vi "UHR-Fleezers Control (host) - 16.2.2v2.vi"() -> ()   [LabVIEW 2014] (continued)
                n1050 = Add(x=w1636, y=w1632) -> (x+y=w1628:dbl)
                n1051 = Greater Or Equal?(x=w1628, y=w1629) -> (x >= y?=w1630:bool)
                n1052 = Select(t=w1629, s=w1630, f=w1628) -> (s? t:f=w1624:dbl)
                n1053 = Index Array(array=w1627, index=1) -> (element=w1625:dbl)
                n1054 = Greater?(x=w1623, y=0) -> (0:w1618:bool)
                n1055 = Greater Or Equal?(x=w1628, y=w1625) -> (x >= y?=w1643:bool)
                n1056 = Select(t=w1618, s="No pause on first pull", f=TRUE ("Scanning (slow scan)")) -> (s? t:f=w1620:bool)
                n1057 = Compound Arithmetic op=AND(w1643, "Stop at pause on pull", w1639, w1620) -> (w1642:bool)
                n1058 = Compound Arithmetic op=OR(w1630, "Immediately quit scan", "Stop pulling and reverse") -> (w1645:bool)
                n1059 = case shown="True" w1642 {
                  tunnel: [w1649 w1651] -> w1640
                  tunnel: w1639 -> [w1649 _]
                  tunnel: w1625 -> [_ w1650]
                  tunnel: w1624 -> [w1648 _]
                  frame False {
                    # "use the current position or the exact position for the final location"
                    n1060 = property on="Trap Delta (MHz)" class="DigNum (strict)"("Val(Sgnl)"=w1648) -> ()  [unwired: 2 in, 2 out]
                  }
                  frame True {
                    # "use the exact postion for the pause"
                    n1061 = while {
                      tunnel: [FALSE] -> w1651
                      i -> [w1662]
                      stop <- w1659 stop-if-true
                      w1663 = u32 100 ("milliseconds to wait")
                      n1062 = local read "Trap pause durations (s)"() -> (w1653:dbl[])
                      n1063 = local read "Immediately quit scan"() -> (w1655:bool)
                      n1064 = Multiply(x="Duration 2 (s)", y=1000.0) -> (x*y=w1664:dbl)
                      n1065 = Divide(x=w1664, y=w1663) -> (x/y=w1661:dbl)
                      n1066 = Wait (ms)(milliseconds to wait=w1663) -> ()  [unwired: 1 out]
                      n1067 = Greater Or Equal?(x=w1662, y=w1661) -> (x >= y?=w1660:bool)
                      n1068 = Or(x="Cancel pause", y=w1655) -> (x .or. y?=w1656:bool)
                      n1069 = Index Array(array=w1653, index=1) -> ()  [unwired: 1 out]
                      n1070 = Or(x=w1660, y=w1656) -> (x .or. y?=w1659:bool)
                    }
                    n1071 = property on="Trap Delta (MHz)" class="DigNum (strict)"("Val(Sgnl)"=w1650) -> ()  [unwired: 2 in, 2 out]
                  }
                }
                "Scanning (slow scan) 2" <- TRUE ("Scanning (slow scan)")
              }
            }
            frame #1 {
              # "Pause between pull/relax"
              # "If you reverse, skip this pause"
              n1072 = Not(x=w1666) -> (.not. x?=w1667:bool)
              n1073 = And(x="Pause after pull, before next relax", y=w1667) -> (x .and. y?=w1668:bool)
              n1074 = case shown="True" w1668 {
                frame False {
                }
                frame True {
                  n1075 = while {
                    i -> [w1679]
                    stop <- w1676 stop-if-true
                    w1680 = u32 100 ("milliseconds to wait")
                    n1076 = local read "Immediately quit scan"() -> (w1673:bool)
                    n1077 = local read "Duration 2 (s)"() -> (w1670:dbl)
                    n1078 = local read "Trap pause durations (s)"() -> (w1671:dbl[])
                    n1079 = local read "Cancel pause"() -> (w1675:bool)
                    n1080 = Multiply(x=w1670, y=1000.0) -> (x*y=w1681:dbl)
                    n1081 = Divide(x=w1681, y=w1680) -> (x/y=w1678:dbl)
                    n1082 = Wait (ms)(milliseconds to wait=w1680) -> ()  [unwired: 1 out]
                    n1083 = Greater Or Equal?(x=w1679, y=w1678) -> (x >= y?=w1677:bool)
                    n1084 = Or(x=w1675, y=w1673) -> (x .or. y?=w1674:bool)
                    n1085 = Index Array(array=w1671, index=2) -> ()  [unwired: 1 out]
                    n1086 = Or(x=w1677, y=w1674) -> (x .or. y?=w1676:bool)
                  }
                }
              }
            }
            frame #2 {
              # "Relax"
              n1087 = while {
                shift-right: [w1702] -> _
                shift-left: TRUE -> [w1701]
                stop <- w1705 stop-if-true
                n1088 = local read "Trap step increment (MHz) (slow scan) 2"() -> (w1696:dbl)
                n1089 = local read "Trap pause positions (MHz)"() -> (w1685:dbl[])
                n1090 = local read "Trap step dwell (ms) (slow scan) 2"() -> (w1692:dbl)
                n1091 = local write "Cancel pause"(FALSE ("Cancel pause")) -> ()
                n1092 = local read "Pause scan"() -> (w1693:bool)
                n1093 = local read "Trap Delta (MHz)"() -> (w1700:dbl)
                n1094 = Index Array(array=w1685, index=0) -> (element=w1689:dbl)
                n1095 = Select(t=0.0, s=w1693, f=w1696) -> (s? t:f=w1695:dbl)
                n1096 = Wait (ms)(milliseconds to wait=w1692) -> ()  [unwired: 1 out]
                n1097 = Subtract(x=w1700, y=w1695) -> (x-y=w1688:dbl)
                n1098 = Less Or Equal?(x=w1688, y=w1689) -> (x <= y?=w1690:bool)
                n1099 = Index Array(array=w1685, index=1) -> (element=w1684:dbl)
                n1100 = local read "Immediately quit scan"() -> (w1699:bool)
                n1101 = Select(t=w1689, s=w1690, f=w1688) -> (s? t:f=w1687:dbl)
                n1102 = Less Or Equal?(x=w1688, y=w1684) -> (x <= y?=w1704:bool)
                n1103 = Compound Arithmetic op=AND(w1704, "Stop at pause on relax", w1701) -> (w1703:bool)
                n1104 = Or(x=w1690, y=w1699) -> (x .or. y?=w1705:bool)
                n1105 = case shown="True" w1703 {
                  tunnel: [w1707 w1709] -> w1702
                  tunnel: w1701 -> [w1707 _]
                  tunnel: w1687 -> [w1706 _]
                  tunnel: w1684 -> [_ w1708]
                  frame False {
                    n1106 = property on="Trap Delta (MHz)" class="DigNum (strict)"("Val(Sgnl)"=w1706) -> ()  [unwired: 2 in, 2 out]
                  }
                  frame True {
                    n1107 = while {
                      tunnel: [FALSE] -> w1709
                      i -> [w1720]
                      stop <- w1717 stop-if-true
                      w1721 = u32 100 ("milliseconds to wait")
                      n1108 = local read "Immediately quit scan"() -> (w1714:bool)
                      n1109 = local read "Trap pause durations (s)"() -> (w1711:dbl[])
                      n1110 = local read "Cancel pause"() -> (w1713:bool)
                      n1111 = local read "Duration 2 (s)"() -> (w1710:dbl)
                      n1112 = Multiply(x=w1710, y=1000.0) -> (x*y=w1722:dbl)
                      n1113 = Divide(x=w1722, y=w1721) -> (x/y=w1719:dbl)
                      n1114 = Wait (ms)(milliseconds to wait=w1721) -> ()  [unwired: 1 out]
                      n1115 = Greater Or Equal?(x=w1720, y=w1719) -> (x >= y?=w1718:bool)
                      n1116 = Or(x=w1713, y=w1714) -> (x .or. y?=w1715:bool)
                      n1117 = Index Array(array=w1711, index=1) -> ()  [unwired: 1 out]
                      n1118 = Or(x=w1718, y=w1715) -> (x .or. y?=w1717:bool)
                    }
                    n1119 = property on="Trap Delta (MHz)" class="DigNum (strict)"("Val(Sgnl)"=w1708) -> ()  [unwired: 2 in, 2 out]
                  }
                }
              }
            }
            frame #3 {
              # "Pause at bottom, after relax, before next pull"
              # "If you reverse, skip this pause"
              n1120 = Increment(x=w1729) -> (x+1=w1731:i32)
              n1121 = Greater Or Equal?(x=w1731, y="Repeat n pull/relax scans") -> (x >= y?=w1733:bool)
              n1122 = local read "Immediately quit scan"() -> (w1732:bool)
              n1123 = Compound Arithmetic op=OR(w1732, w1733, "Finish scan and quit") -> (w1725:bool)
              n1124 = Not(x=w1725) -> (.not. x?=w1724:bool)
              n1125 = And(x="Pause after relax, before next pull", y=w1724) -> (x .and. y?=w1726:bool)
              n1126 = case shown="True" w1726 {
                frame False {
                }
                frame True {
                  n1127 = while {
                    i -> [w1743]
                    stop <- w1740 stop-if-true
                    w1744 = u32 100 ("milliseconds to wait")
                    n1128 = local read "Immediately quit scan"() -> (w1737:bool)
                    n1129 = local read "Duration 2 (s)"() -> (w1734:dbl)
                    n1130 = local read "Trap pause durations (s)"() -> (w1735:dbl[])
                    n1131 = local read "Cancel pause"() -> (w1739:bool)
                    n1132 = Multiply(x=w1734, y=1000.0) -> (x*y=w1745:dbl)
                    n1133 = Divide(x=w1745, y=w1744) -> (x/y=w1742:dbl)
                    n1134 = Wait (ms)(milliseconds to wait=w1744) -> ()  [unwired: 1 out]
                    n1135 = Greater Or Equal?(x=w1743, y=w1742) -> (x >= y?=w1741:bool)
                    n1136 = Or(x=w1739, y=w1737) -> (x .or. y?=w1738:bool)
                    n1137 = Index Array(array=w1735, index=0) -> ()  [unwired: 1 out]
                    n1138 = Or(x=w1741, y=w1738) -> (x .or. y?=w1740:bool)
                  }
                }
              }
            }
          }
          n1139 = Not(x=w1613) -> (.not. x?=w1612:bool)
          n1140 = local write "Scanning (slow scan) 2"(w1612) -> ()
        }
        n1141 = case shown="True" w1554 {
          frame False {
          }
          frame True {
            n1142 = property on="Stop Saving" class="Bool (strict)"("Val(Sgnl)"=TRUE ("Value (Signaling)")) -> ()  [unwired: 2 in, 2 out]
          }
        }
      }
    }
    n1143 = node-c288() -> ()  [unwired: 1 in, 1 out]
  }
  n1144 = timed-loop "Mouse control: trap position (AOM deflection), set confocal spot from image" {
    tunnel: [w1748] -> w92
    timing: w87 -> [_]
    timing-out: [_] -> w86
    tunnel: w36 -> [w1747]
    stop <- w1748 stop-if-true
    n1145 = node-c288() -> ()  [unwired: 2 out]
    n1146 = event shown="[0] \"Pane\": Mouse Down" {
      selector: _ -> [_ _]
      dyn-events: _ -> [_ _]
      timeout: _ -> [_ _]
      tunnel: w1747 -> [w1751 _]
      event Mouse Down {
        n1147 = event-data() -> ("Time"=w1753:u32, "Coords"=w1752:T9, "Button"=w1754:u16)  [unwired: 6 out]
        n1148 = case shown="3" w1754 {
          tunnel: w1753 -> [_ _ w1860]
          tunnel: w1752 -> [_ w1791 w1858]
          tunnel: w1751 -> [_ _ w1854]
          frame 0, Default {
          }
          frame 1 {
            n1149 = property on="APD 2" class="ImageControl"() -> ("Displayed Image Position"=w1761:cluster{"Left":i32, "Top":i32})  [unwired: 2 in, 2 out]
            n1150 = property on="APD 1" class="ImageControl"() -> ("Displayed Image Position"=w1790:cluster{"Left":i32, "Top":i32})  [unwired: 2 in, 2 out]
            n1151 = property on="Detection Laser X" class="ImageControl"() -> ("Displayed Image Position"=w1787:cluster{"Left":i32, "Top":i32})  [unwired: 2 in, 2 out]
            n1152 = property on="Detection Laser Y" class="ImageControl"() -> ("Displayed Image Position"=w1786:cluster{"Left":i32, "Top":i32})  [unwired: 2 in, 2 out]
            n1153 = property on="APD 2" class="ImageControl"() -> ("Displayed Image Size"=w1760:cluster{"Width":u32, "Height":u32})  [unwired: 2 in, 2 out]
            n1154 = property on="APD 1" class="ImageControl"() -> ("Displayed Image Size"=w1788:cluster{"Width":u32, "Height":u32})  [unwired: 2 in, 2 out]
            n1155 = property on="Detection Laser X" class="ImageControl"() -> ("Displayed Image Size"=w1789:cluster{"Width":u32, "Height":u32})  [unwired: 2 in, 2 out]
            n1156 = property on="Detection Laser Y" class="ImageControl"() -> ("Displayed Image Size"=w1785:cluster{"Width":u32, "Height":u32})  [unwired: 2 in, 2 out]
            n1157 = Unbundle By Name(w1760) -> ("Width"=w1757:u32, "Height"=w1756:u32)
            n1158 = Unbundle By Name(w1761) -> ("Left"=w1759:i32, "Top"=w1758:i32)
            n1159 = Unbundle By Name(w1788) -> ("Width"=w1782:u32, "Height"=w1781:u32)
            n1160 = Unbundle By Name(w1789) -> ("Width"=w1778:u32, "Height"=w1777:u32)
            n1161 = Unbundle By Name(w1785) -> ("Width"=w1774:u32, "Height"=w1773:u32)
            n1162 = Unbundle By Name(w1790) -> ("Left"=w1784:i32, "Top"=w1783:i32)
            n1163 = Unbundle By Name(w1787) -> ("Left"=w1780:i32, "Top"=w1779:i32)
            n1164 = Unbundle By Name(w1786) -> ("Left"=w1776:i32, "Top"=w1775:i32)
            n1165 = Bundle("Left"=w1759, "Top"=w1758, "Width"=w1757, "Height"=w1756) -> (w1755:T36)  [unwired: 1 in]
            n1166 = Bundle("Left"=w1784, "Top"=w1783, "Width"=w1782, "Height"=w1781) -> (w1772:T36)  [unwired: 1 in]
            n1167 = Bundle("Left"=w1780, "Top"=w1779, "Width"=w1778, "Height"=w1777) -> (w1771:T36)  [unwired: 1 in]
            n1168 = Bundle("Left"=w1776, "Top"=w1775, "Width"=w1774, "Height"=w1773) -> (w1770:T36)  [unwired: 1 in]
            n1169 = Build Cluster Array(w1755, w1772, w1771, w1770) -> (w1769:T37)
            n1170 = for {
              tunnel: w1791 -> [w1802]
              tunnel: w1769 -> [w1803] mode=indexing
              shift-right: [w1800] -> w1767
              shift-left: TRUE -> [w1801]
              shift-right: [w1799] -> w1765
              shift-left: _ -> [w1795]
              shift-right: [w1798] -> w1764
              shift-left: _ -> [w1794]
              shift-right: [w1797] -> w1763
              shift-left: _ -> [w1793]
              shift-right: [w1796] -> w1762
              shift-left: _ -> [w1792]
              n1171 = case shown="True" w1801 {
                selector: w1801 -> [w1808 _]
                tunnel: w1803 -> [_ w1817]
                tunnel: w1802 -> [_ w1815]
                tunnel: [w1808 w1813] -> w1800
                tunnel: [w1807 w1812] -> w1799
                tunnel: [w1806 w1811] -> w1798
                tunnel: [w1805 w1810] -> w1797
                tunnel: [w1804 w1809] -> w1796
                tunnel: w1795 -> [w1807 _]
                tunnel: w1794 -> [w1806 _]
                tunnel: w1793 -> [w1805 _]
                tunnel: w1792 -> [w1804 _]
                frame False {
                }
                frame True {
                  n1172 = Unbundle(w1817) -> (w1816:T36)
                  n1173 = call "isclickinwindow.vi"("Image Param"=w1816, "Point32"=w1815) -> ("4 Y"=w1809:i32, "3 Height"=w1810:i32, "2 X"=w1811:i32, "1 Width"=w1812:i32, "In image?"=w1814:bool)  [unwired: 1 in]
                  n1174 = Not(x=w1814) -> (.not. x?=w1813:bool)
                }
              }
            }
            n1175 = Not(x=w1767) -> (.not. x?=w1766:bool)
            n1176 = case shown="True" w1766 {
              tunnel: w1764 -> [_ w1831]
              tunnel: w1762 -> [_ w1830]
              tunnel: w1765 -> [_ w1829]
              tunnel: w1763 -> [_ w1828]
              frame False {
              }
              frame True {
                w1818 = FALSE ("Get Point")
                n1177 = local read "Scan lines (y)"() -> (w1833:u64)
                n1178 = disable-structure shown="Disabled" {
                  frame Disabled {
                  }
                  frame Enabled {
                  }
                }
                n1179 = local read "Actual MCL Inc (V)"() -> (w1827:dbl)
                n1180 = local read "Scan steps (MCL)"() -> (w1832:u64)
                n1181 = Divide "Y Pix/step"(x=w1828, y=w1833) -> (x/y=w1840:dbl)
                n1182 = Divide "Y V/pix"(x=w1827, y=w1840) -> (x/y=w1839:dbl)
                n1183 = Divide "Y half step offset"(x=w1827, y=2.0) -> (x/y=w1841:dbl)
                n1184 = Divide "X pix/step"(x=w1829, y=w1832) -> (x/y=w1838:dbl)
                n1185 = Negate(x=w1841) -> (-x=w1842:dbl)
                n1186 = local read "Initial Y"() -> (w1848:dbl)
                n1187 = Multiply(x=w1830, y=w1839) -> (x*y=w1849:dbl)
                n1188 = Divide "X half step offset"(x=w1827, y=2.0) -> (x/y=w1835:dbl)
                n1189 = Divide "X V/pix"(x=w1827, y=w1838) -> (x/y=w1837:dbl)
                n1190 = Multiply(x=w1827, y=w1832) -> (x*y=w1844:dbl)
                n1191 = Compound Arithmetic op=ADD(w1842, w1849, w1848) -> (w1819:dbl)
                "Pointer Y (V)" <- w1819
                n1192 = Multiply(x=w1837, y=w1831) -> (x*y=w1846:dbl)
                n1193 = Negate(x=w1835) -> (-x=w1834:dbl)
                n1194 = local read "Initial X"() -> (w1847:dbl)
                n1195 = Negate(x=w1846) -> (-x=w1845:dbl)
                n1196 = Compound Arithmetic op=ADD(w1834, w1844, w1847, w1845) -> (w1820:dbl)
                "Pointer X (V)" <- w1820
                n1197 = case shown="True" "Set High F Confocal Spot (X-Y)" {
                  tunnel: w1820 -> [_ w1850]
                  tunnel: w1819 -> [_ w1851]
                  frame False {
                  }
                  frame True {
                    "Confocal Y 2 (V)" <- w1851
                    "Confocal X 2 (V)" <- w1850
                  }
                }
                n1198 = Or(x="Set X Only", y="Set Confocal Spot (X-Y)") -> (x .or. y?=w1823:bool)
                n1199 = Or(x="Set Confocal Spot (X-Y)", y="Set Y Only") -> (x .or. y?=w1822:bool)
                n1200 = case shown="True" w1823 {
                  tunnel: w1820 -> [_ w1852]
                  frame False {
                  }
                  frame True {
                    n1201 = property on="AO2" class="Slide (strict)"("Val(Sgnl)"=w1852) -> ()  [unwired: 2 in, 2 out]
                    "Confocal X 1 (V)" <- w1852
                  }
                }
                n1202 = case shown="True" w1822 {
                  tunnel: w1819 -> [_ w1853]
                  frame False {
                  }
                  frame True {
                    n1203 = property on="AO1" class="Slide (strict)"("Val(Sgnl)"=w1853) -> ()  [unwired: 2 in, 2 out]
                    "Confocal Y 1 (V)" <- w1853
                  }
                }
                n1204 = local write "Set High F Confocal Spot (X-Y)"(w1818) -> ()
                n1205 = local write "Set Confocal Spot (X-Y)"(w1818) -> ()
                n1206 = local write "Set X Only"(w1818) -> ()
                n1207 = local write "Set Y Only"(w1818) -> ()
              }
            }
          }
          frame 3 {
            n1208 = local read "BD 2 Frequency 1 (MHz)"() -> (w1855:dbl)
            n1209 = local read "BD 1 Frequency 1 (MHz)"() -> (w1856:dbl)
            n1210 = local write "Manipulating Trap"(TRUE ("Manipulating Trap")) -> ()
            n1211 = local write "Coords"(T9 {"Horizontal"=0, "Vertical"=0} ("Coords")) -> ()
            n1212 = while {
              tunnel: w1860 -> [w1865]
              tunnel: w1858 -> [w1864]
              tunnel: w1856 -> [w1863]
              tunnel: w1855 -> [w1862]
              tunnel: w1854 -> [w1861]
              stop <- w1866 stop-if-true
              n1213 = event shown="[0] \"Pane\": Mouse Move" {
                selector: _ -> [_ _]
                dyn-events: _ -> [_ _]
                timeout: _ -> [_ _]
                tunnel: ["Force Manip Abort" w1933] -> w1866
                tunnel: w1865 -> [w1873 _]
                tunnel: w1864 -> [w1871 _]
                tunnel: w1863 -> [w1870 _]
                tunnel: w1862 -> [w1869 _]
                tunnel: w1861 -> [w1867 _]
                event Mouse Move {
                  n1214 = event-data() -> ("Time"=w1874:u32, "Coords"=w1875:T9)  [unwired: 3 out]
                  n1215 = Less?(x=w1874, y=w1873) -> (x < y?=w1872:bool)
                  n1216 = case "Makes sure old motion events prior to mouse click aren't used" shown="False" w1872 {
                    tunnel: w1875 -> [w1920 _]
                    tunnel: w1871 -> [w1921 _]
                    tunnel: w1870 -> [w1896 _]
                    tunnel: w1869 -> [w1895 _]
                    tunnel: w1867 -> [w1880 _]
                    frame False {
                      n1217 = Subtract(x=w1920, y=w1921) -> (x-y=w1919:T9)
                      "Coords" <- w1919
                      n1218 = local read "Y RF Frequency Limits (MHz)"() -> (w1881:T18)
                      n1219 = To Double Precision Float(number=w1919) -> (double precision float=w1918:cluster{"Horizontal":dbl, "Vertical":dbl})
                      n1220 = Multiply(x=cluster{"Horizontal":dbl, "Vertical":dbl} {"Horizontal"=-1.0, "Vertical"=1.0}, y="Manipulation Scaling") -> (x*y=w1914:cluster{"Horizontal":dbl, "Vertical":dbl})
                      n1221 = local read "X RF Frequency Limits (MHz)"() -> (w1882:T18)
                      n1222 = Multiply(x=w1918, y=w1914) -> (x*y=w1916:cluster{"Horizontal":dbl, "Vertical":dbl})
                      n1223 = Unbundle By Name(w1916) -> ("Horizontal"=w1911:dbl, "Vertical"=w1915:dbl)
                      n1224 = Unbundle By Name(w1881) -> ("Maximum"=w1884:dbl, "Minimum"=w1883:dbl)
                      n1225 = Boolean To (0,1)(Boolean="Manip. X?") -> (0, 1=w1909:i16)
                      n1226 = Boolean To (0,1)(Boolean="Manip. Y?") -> (0, 1=w1906:i16)
                      n1227 = local read "BD 1 Frequency 2 (MHz)"() -> (w1898:dbl)
                      n1228 = Multiply(x=w1915, y=w1906) -> (x*y=w1908:dbl)
                      n1229 = Multiply(x=w1909, y=w1911) -> (x*y=w1912:dbl)
                      n1230 = local read "BD 2 Frequency 2 (MHz)"() -> (w1897:dbl)
                      n1231 = Unbundle By Name(w1882) -> ("Maximum"=w1886:dbl, "Minimum"=w1885:dbl)
                      n1232 = Add(x=w1895, y=w1908) -> (x+y=w1888:dbl)
                      n1233 = Add(x=w1896, y=w1912) -> (x+y=w1890:dbl)
                      n1234 = In Range and Coerce(upper limit=w1886, x=w1890, lower limit=w1885) -> (coerced(x)=w1889:dbl)  [unwired: 1 out]
                      n1235 = In Range and Coerce(upper limit=w1884, x=w1888, lower limit=w1883) -> (coerced(x)=w1887:dbl)  [unwired: 1 out]
                      n1236 = Subtract(x=w1887, y=w1897) -> (x-y=w1904:dbl)
                      n1237 = Subtract(x=w1889, y=w1898) -> (x-y=w1905:dbl)
                      n1238 = local read "Ignore BD 2 for trap delta"() -> (w1877:bool)
                      n1239 = Square(x=w1904) -> (x^2=w1879:dbl)
                      n1240 = Square(x=w1905) -> (x^2=w1903:dbl)
                      n1241 = Select(t=0.0, s=w1877, f=w1879) -> (s? t:f=w1878:dbl)
                      n1242 = Add(x=w1903, y=w1878) -> (x+y=w1902:dbl)
                      n1243 = Square Root(x=w1902) -> (sqrt(x)=w1899:dbl)
                      n1244 = In Range and Coerce(upper limit="Limit Max (MHz)", x=w1899, lower limit="Limit Min (MHz)") -> (In Range?=w1892:bool)  [unwired: 1 out]
                      n1245 = Not(x="Limits Enable") -> (.not. x?=w1891:bool)
                      n1246 = Or(x=w1892, y=w1891) -> (x .or. y?=w1893:bool)
                      n1247 = case shown="True" w1893 {
                        tunnel: w1899 -> [_ w1923]
                        tunnel: w1889 -> [_ w1930]
                        tunnel: w1898 -> [_ w1929]
                        tunnel: w1887 -> [_ w1928]
                        tunnel: w1897 -> [_ w1927]
                        tunnel: w1882 -> [_ w1925]
                        tunnel: w1881 -> [_ w1924]
                        tunnel: w1880 -> [_ w1922]
                        frame False {
                        }
                        frame True {
                          n1248 = local read "BD 1 Frequency 3 (MHz)"() -> (w1931:dbl)
                          n1249 = local read "BD 2 Frequency 3 (MHz)"() -> (w1926:dbl)
                          n1250 = local write "Trap Delta (MHz)"(w1923) -> ()
                          n1251 = call "set RF board frequency - interlace.vi"("Board 2 Frequency Limits"=w1924, "Board 1 Frequency Limits"=w1925, "FPGA VI Reference In"=w1922, "Board 2 Frequency 3 (MHz)"=w1926, "Board 1 Frequency 3 (MHz)"=w1931, "Board 2 Frequency 2 (MHz)"=w1927, "Board 2 Frequency 1 (MHz)"=w1928, "Board 1 Frequency 2 (MHz)"=w1929, "Board 1 Frequency 1  (MHz)"=w1930) -> ()  [unwired: 1 in, 2 out]
                          n1252 = local write "BD 2 Frequency 1 (MHz)"(w1928) -> ()
                          n1253 = local write "BD 1 Frequency 1 (MHz)"(w1930) -> ()
                        }
                      }
                    }
                    frame True {
                    }
                  }
                }
                event Mouse Up {
                  n1254 = event-data() -> ("Button"=w1932:u16)  [unwired: 8 out]
                  n1255 = case shown="3" w1932 {
                    tunnel: [FALSE TRUE] -> w1933
                    frame 0, Default {
                    }
                    frame 3 {
                      n1256 = local read "Trap Delta (MHz)"() -> (w1935:dbl)
                      n1257 = property on="Initial delta (MHz)" class="DigNum (strict)"("Val(Sgnl)"=w1935) -> ()  [unwired: 2 in, 2 out]
                      n1258 = local write "Manipulating Trap"(FALSE ("Manipulating Trap")) -> ()
                    }
                  }
                }
              }
            }
          }
        }
      }
      event Mouse Move {
        n1259 = event-data() -> ()  [unwired: 6 out]
      }
    }
    n1260 = local read "Stop All"() -> (w1748:bool)
    n1261 = node-c288() -> ()  [unwired: 2 out]
  }
  n1262 = timed-loop "Rough control of MCL mirror stage (debugging)" {
    tunnel: [w1940] -> w94
    timing: w46 -> [_]
    timing-out: [_] -> w45
    tunnel: w36 -> [w1938]
    stop <- w1940 stop-if-true
    n1263 = node-c288() -> ()  [unwired: 2 out]
    n1264 = case shown="2" "MCL Mode" {
      tunnel: w1938 -> [_ w1943 w1990]
      frame 0, Default {
      }
      frame 1 {
        n1265 = node-c288() -> (w1945:T28)  [unwired: 4 out]
        n1266 = timed-loop "Oscillate MCL mirror" {
          timing: w1945 -> [_]
          timing-out: [_] -> w1944
          tunnel: w1943 -> [w1946]
          i -> [w1984]
          stop <- w1947 stop-if-true
          n1267 = node-c288() -> (w1983:i64)  [unwired: 1 out]
          n1268 = Multiply(x="AO1", y=32767.0) -> (x*y=w1979:dbl)
          n1269 = Multiply(x="AO2", y=32767.0) -> (x*y=w1974:dbl)
          n1270 = Divide(x=w1979, y=10.0) -> (x/y=w1980:dbl)
          n1271 = Divide(x=w1974, y=10.0) -> (x/y=w1975:dbl)
          n1272 = To Word Integer(number=w1980) -> (16bit integer=w1972:i16)
          n1273 = To Word Integer(number=w1975) -> (16bit integer=w1971:i16)
          n1274 = Divide(x=w1983, y=i64 1000) -> (x/y=w1954:dbl)
          n1275 = Multiply(x=w1954, y=w1984) -> (x*y=w1965:dbl)
          n1276 = Multiply(x="Osc. freq. (Hz) 2", y=6.283185307179586) -> (x*y=w1966:dbl)
          n1277 = Multiply(x=w1966, y=w1965) -> (x*y=w1964:dbl)
          n1278 = Sine(x=w1964) -> (sin(x)=w1963:dbl)
          n1279 = Multiply(x=w1963, y="Osc. amp. (V)") -> (x*y=w1961:dbl)
          n1280 = Add(x=w1961, y="Osc. center (V)") -> (x+y=w1959:dbl)
          n1281 = Divide(x=w1959, y=10.0) -> (x/y=w1957:dbl)
          n1282 = Multiply(x=w1957, y=32767.0) -> (x*y=w1952:dbl)
          n1283 = Select(t=w1952, s="Scan axis", f=w1972) -> (s? t:f=w1970:dbl)
          n1284 = Select(t=w1971, s="Scan axis", f=w1952) -> (s? t:f=w1969:dbl)
          n1285 = local read "MCL Mode"() -> (w1951:u16)
          n1286 = Not Equal?(x=w1951, y=u16 1) -> (x != y?=w1948:bool)
          n1287 = local read "Stop All"() -> (w1949:bool)
          n1288 = xnode "Read/Write Control"("FPGA VI Reference In"=w1946, "AO1"=w1970, "AO2"=w1969) -> ()  [unwired: 1 in, 2 out]
          n1289 = Compound Arithmetic op=OR(w1949, w1948) -> (w1947:bool)
          n1290 = node-c288() -> ()  [unwired: 2 out]
        }
        n1291 = node-c288(w1944) -> ()  [unwired: 1 out]
      }
      frame 2 {
        n1292 = case shown="True" "Start Scan" {
          tunnel: w1990 -> [_ w1992]
          frame False {
          }
          frame True {
            n1293 = Subtract(x="End (V)", y="Begin (V)") -> (x-y=w1999:dbl)
            n1294 = Decrement(x="N Points") -> (x-1=w1998:dbl)
            n1295 = Divide(x=w1999, y=w1998) -> (x/y=w1996:dbl)
            n1296 = for {
              N: "N Points" -> [_]
              tunnel: "Begin (V)" -> [w2015]
              tunnel: [w2007] -> w2002 mode=indexing
              tunnel: w1996 -> [w2006]
              tunnel: [w2004] -> w1995 mode=indexing
              tunnel: w1992 -> [w2003]
              i -> [w2014]
              n1297 = Multiply(x=w2006, y=w2014) -> (x*y=w2013:dbl)
              n1298 = Add(x=w2015, y=w2013) -> (x+y=w2010:dbl)
              n1299 = local read "Scan axis"() -> (w2005:bool)
              n1300 = local read "AO1"() -> (w2012:dbl)
              n1301 = local read "AO2"() -> (w2011:dbl)
              n1302 = Select(t=w2010, s=w2005, f=w2012) -> (s? t:f=w2009:dbl)
              n1303 = Select(t=w2011, s=w2005, f=w2010) -> (s? t:f=w2008:dbl)
              n1304 = flat-sequence {
                tunnel: w2009 -> [w2019]
                tunnel: w2008 -> [w2018]
                tunnel: w2003 -> [w2016]
                tunnel: [w2029] -> w2007
                tunnel: [w2028] -> w2004
                frame #0 {
                  w2022 = 10.0 ("y")
                  w2017 = 32767.0 ("y")
                  n1305 = Multiply(x=w2019, y=w2017) -> (x*y=w2025:dbl)
                  n1306 = Multiply(x=w2018, y=w2017) -> (x*y=w2023:dbl)
                  n1307 = Divide(x=w2025, y=w2022) -> (x/y=w2026:dbl)
                  n1308 = Divide(x=w2023, y=w2022) -> (x/y=w2024:dbl)
                  n1309 = To Word Integer(number=w2026) -> (16bit integer=w2020:i16)
                  n1310 = To Word Integer(number=w2024) -> (16bit integer=w2021:i16)
                  n1311 = xnode "Read/Write Control"("FPGA VI Reference In"=w2016, "AO1"=w2020, "AO2"=w2021) -> ()  [unwired: 1 in, 2 out]
                }
                frame #1 {
                  n1312 = Wait (ms)(milliseconds to wait="DAQ Delay (ms)") -> ()  [unwired: 1 out]
                }
                frame #2 {
                  n1313 = local read "Slow mean"() -> (w2029:dbl)
                  n1314 = local read "Sigma"() -> (w2028:dbl)
                }
              }
            }
            n1315 = Bundle("Begin (V)"="Begin (V)", w1996, w2002) -> (→"MCL Scan":cluster{"Begin (V)":dbl, dbl, dbl[]})  [unwired: 1 out]
            n1316 = Bundle("Begin (V)"="Begin (V)", w1996, w1995) -> (→"MCL Scan 2":cluster{"Begin (V)":dbl, dbl, dbl[]})  [unwired: 1 out]
          }
        }
      }
    }
    n1317 = local read "Stop All"() -> (w1940:bool)
    n1318 = node-c288() -> ()  [unwired: 2 out]
  }
  n1319 = timed-loop "Oscillate Trap/AOM (fishing, conjugate plane alignment)" {
    tunnel: [w2032] -> w88
    timing: w83 -> [_]
    timing-out: [_] -> w82
    tunnel: w36 -> [w2031]
    tunnel: w15 -> [w2030]
    stop <- w2032 stop-if-true
    n1320 = node-c288() -> ()  [unwired: 2 out]
    n1321 = event shown="[0] \"Oscillate Set 1\", \"Fish for Tether\": Value Change" {
      selector: _ -> [_ _ _ _]
      dyn-events: _ -> [_ _ _ _]
      timeout: _ -> [_ _ _ _]
      tunnel: [FALSE ("Stop All") _ _ w2703] -> w2032
      tunnel: w2031 -> [w2035 _ _ _]
      tunnel: w2030 -> [_ _ w2640 _]
      event "Oscillate Set 1", "Fish for Tether": Value Change {
        n1322 = event-data() -> ()  [unwired: 6 out]
        n1323 = local read "Oscillate Set 1"() -> (w2039:bool)
        n1324 = Or(x=w2039, y="Fish for Tether") -> (x .or. y?=w2037:bool)
        n1325 = case shown="True" w2037 {
          tunnel: "Fish for Tether" -> [_ w2042]
          tunnel: w2035 -> [_ w2040]
          frame False {
          }
          frame True {
            n1326 = case shown="True" w2042 {
              selector: w2042 -> [w2045 w2051]
              tunnel: [w2045 w2051] -> w2041
              frame False {
              }
              frame True {
                n1327 = local write "Scan axis 2"(TRUE) -> ()
                n1328 = local write "Tether"(FALSE ("Tether")) -> ()
                n1329 = local read "Flow ON during cal?"() -> (w2046:bool)
                n1330 = property on="Trap Delta (MHz)" class="DigNum (strict)"("Val(Sgnl)"="Furthest Delta (MHz)") -> ()  [unwired: 2 in, 2 out]
                n1331 = Or(x="Flow ON during \nfishing?", y=w2046) -> (x .or. y?=w2047:bool)
                n1332 = Wait (ms)(milliseconds to wait=u32 500) -> ()  [unwired: 1 out]
                n1333 = property on="Sample Channel\nFlow" class="Bool (strict)"("Val(Sgnl)"=w2047) -> ()  [unwired: 2 in, 2 out]
              }
            }
            n1334 = node-c288() -> (w2044:T28)  [unwired: 1 in, 3 out]
            n1335 = timed-loop "Oscillate AOD" {
              timing: w2044 -> [_]
              timing-out: [_] -> w2043
              tunnel: w2041 -> [w2055]
              tunnel: w2040 -> [w2054]
              i -> [w2063]
              stop <- w2061 stop-if-true
              n1336 = node-c288() -> (w2062:i64)  [unwired: 1 out]
              n1337 = flat-sequence {
                tunnel: w2063 -> [w2090]
                tunnel: w2062 -> [w2089]
                tunnel: w2055 -> [w2073]
                tunnel: [w2073] -> w2060
                tunnel: [w2072] -> w2059
                tunnel: [w2071] -> w2058
                tunnel: [w2068] -> w2056
                tunnel: w2054 -> [w2064]
                tunnel: w2060 -> [w2137]
                tunnel: w2059 -> [w2135]
                tunnel: w2058 -> [w2134]
                tunnel: [w2133] -> w2057
                tunnel: w2056 -> [w2132]
                tunnel: [w2209] -> w2061
                tunnel: w2057 -> [w2208]
                frame #0 {
                  # "w (rad/s)"
                  # "t (s)"
                  n1338 = Divide(x=w2089, y=i64 1000) -> (x/y=w2065:dbl)
                  n1339 = local read "BD 1 Frequency 2 (MHz)"() -> (w2067:dbl)
                  n1340 = Multiply(x="Osc. freq. (Hz)", y=6.283185307179586) -> (x*y=w2087:dbl)
                  n1341 = Multiply(x=w2065, y=w2090) -> (x*y=w2086:dbl)
                  n1342 = Multiply(x=w2087, y=w2086) -> (x*y=w2070:dbl)
                  n1343 = local read "BD 1 Frequency 1 (MHz)"() -> (w2075:dbl)
                  n1344 = case shown="True" w2073 {
                    tunnel: w2070 -> [w2096 w2115]
                    tunnel: w2075 -> [_ w2123]
                    tunnel: w2067 -> [_ w2124]
                    tunnel: [w2093 w2119] -> w2066
                    tunnel: [FALSE w2097] -> w2071
                    tunnel: [0.0 w2111] -> w2068
                    frame False {
                      n1345 = Sine(x=w2096) -> (sin(x)=w2094:dbl)
                      n1346 = Multiply(x=w2094, y="Osc. amp. (MHz)") -> (x*y=w2093:dbl)
                    }
                    frame True {
                      # "trap position goes from 0 to 1 (0 is when it is furthest away, 1 is when closest)\nso we want to test for tether only when farther away, or x < 1"
                      # "quit if taking too long"
                      # "oscillate the trap"
                      # "Test for tether"
                      n1347 = local read "Vec Mean of T1 T2"() -> (w2100:dbl[])
                      "Trigger Signal" <- w2100
                      n1348 = Cosine(x=w2115) -> (cos(x)=w2127:dbl)
                      n1349 = Subtract(x=w2124, y=w2123) -> (x-y=w2122:dbl)
                      n1350 = Decrement(x=w2127) -> (x-1=w2126:dbl)
                      n1351 = Subtract(x=w2122, y="Closest Delta (MHz)") -> (x-y=w2120:dbl)
                      n1352 = Divide(x=w2126, y=-2.0) -> (x/y=w2110:dbl)
                      n1353 = Greater?(x=w2100, y="Stop F (pN)") -> (0:w2117:bool[])
                      n1354 = Multiply(x=w2110, y=w2120) -> (x*y=w2119:dbl)
                      n1355 = Less?(x=w2110, y="Fish mask thresh") -> (x < y?=w2109:bool)
                      n1356 = Boolean To (0,1)(Boolean=w2109) -> (0, 1=w2107:i16)
                      n1357 = Multiply(x=w2107, y=w2100) -> (x*y=w2106:dbl[])
                      n1358 = Divide(x=w2115, y=6.283185307179586) -> (x/y=w2114:dbl)
                      n1359 = Round Toward +Infinity(x=w2114) -> (ceil(x): smallest int >= x=w2111:dbl)
                      "Attempts" <- w2111
                      n1360 = Greater?(x=w2106, y="Stop F (pN) (mask)") -> (0:w2104:bool[])
                      n1361 = Or Array Elements(Boolean array=w2117) -> (logical OR=w2102:bool)
                      n1362 = Or Array Elements(Boolean array=w2104) -> (logical OR=w2101:bool)
                      n1363 = Greater?(x=w2111, y="Attempt Limit") -> (0:w2113:bool)
                      n1364 = case shown="True" w2113 {
                        frame False {
                        }
                        frame True {
                          n1365 = local write "Fish for Tether"(FALSE ("Fish for Tether")) -> ()
                          n1366 = call <vilib>:"Beep.vi"() -> ()  [unwired: 3 in, 9 out]
                          n1367 = local read "Messages"() -> (w2129:string)
                          n1368 = call "Update messages.vi"("Message to add"="Tether fishing timeout." ("Messages"), "Old message string"=w2129) -> ("New message string"=→"Messages":string)
                        }
                      }
                      n1369 = Select(t=w2102, s="Normal (on) or masked test (off)", f=w2101) -> (s? t:f=w2099:bool)
                      n1370 = And(x="Stop Fishing When Tether", y=w2099) -> (x .and. y?=w2097:bool)
                    }
                  }
                  n1371 = local read "BD 2 Frequency 1 (MHz)"() -> (w2074:dbl)
                  n1372 = Select(t=w2075, s="Scan axis 2", f=w2074) -> (s? t:f=w2078:dbl)
                  n1373 = Add(x=w2066, y=w2078) -> (x+y=w2072:dbl)
                  n1374 = Select(t=w2072, s="Scan axis 2", f=w2075) -> (s? t:f=w2081:dbl)
                  n1375 = Select(t=w2074, s="Scan axis 2", f=w2072) -> (s? t:f=w2080:dbl)
                  n1376 = local read "BD 2 Frequency 2 (MHz)"() -> (w2083:dbl)
                  n1377 = local read "BD 2 Frequency 3 (MHz)"() -> (w2082:dbl)
                  n1378 = local read "Y RF Frequency Limits (MHz)"() -> (w2076:T18)
                  n1379 = local read "X RF Frequency Limits (MHz)"() -> (w2077:T18)
                  n1380 = local read "BD 1 Frequency 3 (MHz)"() -> (w2084:dbl)
                  n1381 = call "set RF board frequency - interlace.vi"("Board 2 Frequency Limits"=w2076, "Board 1 Frequency Limits"=w2077, "FPGA VI Reference In"=w2064, "Board 2 Frequency 3 (MHz)"=w2082, "Board 1 Frequency 3 (MHz)"=w2084, "Board 2 Frequency 2 (MHz)"=w2083, "Board 2 Frequency 1 (MHz)"=w2080, "Board 1 Frequency 2 (MHz)"=w2067, "Board 1 Frequency 1  (MHz)"=w2081) -> ()  [unwired: 1 in, 2 out]
                }
                frame #1 {
                  n1382 = And(x=w2137, y=w2134) -> (x .and. y?=w2136:bool)
                  n1383 = case "Only if were fishing and now formed tether" shown="True" w2136 {
                    tunnel: w2135 -> [w2139 w2154]
                    tunnel: [w2138 w2153] -> w2133
                    tunnel: w2132 -> [_ w2149]
                    frame False {
                      n1384 = local read "Fish for Tether"() -> (w2138:bool)
                      n1385 = case shown="False" w2138 {
                        tunnel: w2139 -> [w2140 _]
                        frame False {
                          n1386 = property on="BD 1 Frequency 1 (MHz)" class="DigNum (strict)"("Val(Sgnl)"=w2140) -> ()  [unwired: 2 in, 2 out]
                        }
                        frame True {
                        }
                      }
                    }
                    frame True {
                      w2153 = FALSE ("Fish for Tether")
                      n1387 = call <vilib>:"Beep.vi"() -> ()  [unwired: 3 in, 9 out]
                      n1388 = Number To Decimal String(number=w2149, width (-)=i16 1) -> (decimal integer string=w2147:string)
                      n1389 = Concatenate Strings("Formed tether in ", w2147, " attempt(s)." ("string")) -> (w2144:string)
                      n1390 = local read "Messages"() -> (w2151:string)
                      n1391 = local write "Fish for Tether"(w2153) -> ()
                      n1392 = call "Update messages.vi"("Message to add"=w2144, "Old message string"=w2151) -> ("New message string"=w2150:string)
                      n1393 = local write "Messages"(w2150) -> ()
                      n1394 = Get Date/Time In Seconds() -> (seconds since 1Jan1904=→"Time tether formed":timestamp)
                      n1395 = local read "Flow ON during cal?"() -> (w2141:bool)
                      n1396 = property on="Sample Channel\nFlow" class="Bool (strict)"("Val(Sgnl)"=w2141) -> (error out=w2142:errorcluster)  [unwired: 2 in, 1 out]
                      n1397 = case shown="\"2\", \"3\", \"4\", \"5\", \"6\"" "Then..." {
                        selector: "Then..." -> [_ w2157]
                        tunnel: w2154 -> [w2156 _]
                        tunnel: w2142 -> [_ _]
                        frame "1", Default {
                          n1398 = property on="BD 1 Frequency 1 (MHz)" class="DigNum (strict)"("Val(Sgnl)"=w2156) -> ()  [unwired: 2 in, 2 out]
                        }
                        frame "2", "3", "4", "5", "6" {
                          n1399 = flat-sequence {
                            tunnel: w2157 -> [w2159]
                            frame #0 {
                              n1400 = property on="Trap Delta (MHz)" class="DigNum (strict)"("Val(Sgnl)"="Move to Delta 1 (MHz)") -> ()  [unwired: 2 in, 2 out]
                            }
                            frame #1 {
                              n1401 = case shown="\"5\", \"6\"" w2159 {
                                selector: w2159 -> [w2162 w2172 _]
                                frame "3", "4" {
                                n1402 = flat-sequence {
                                tunnel: w2162 -> [w2163]
                                tunnel: [w2163] -> w2160
                                tunnel: [w2165] -> w2161
                                tunnel: w2160 -> [w2165]
                                tunnel: w2161 -> [w2169]
                                frame #0 {
                                n1403 = property on="Green Laser ON" class="Bool (strict)"("Val(Sgnl)"=TRUE ("Value (Signaling)")) -> ()  [unwired: 2 in, 2 out]
                                }
                                frame #1 {
                                n1404 = Multiply(x="Wait Before Save (s)", y=u32 1000 ("x")) -> (x*y=w2167:u32)
                                n1405 = Wait (ms)(milliseconds to wait=w2167) -> ()  [unwired: 1 out]
                                }
                                frame #2 {
                                n1406 = property on="Start Saving" class="Bool (strict)"("Value"=TRUE ("Start Saving")) -> ()  [unwired: 2 in, 2 out]
                                n1407 = case shown="\"4\"" w2169 {
                                frame Default {
                                }
                                frame "4" {
                                n1408 = property on="Fl. Triggered..." class="Bool (strict)"("Val(Sgnl)"=TRUE ("Value (Signaling)")) -> ()  [unwired: 2 in, 2 out]
                                }
                                }
                                }
                                }
                                }
                                frame "5", "6" {
                                n1409 = stacked-sequence {
                                tunnel: w2172 -> [_ _ _ _ _ _ w2184]
                                frame #0 {
                                n1410 = Replace Array Subset(array=u32[] [0] ("Index Values"), new element="Raster Set Upon Tether", index=0) -> (w2173:u32[])
                                n1411 = property on="Saved AOD Raster Scan Parameter Sets" class="Arr (strict)"("Index Values"=w2173) -> ()  [unwired: 2 in, 2 out]
                                }
                                frame #1 {
                                n1412 = Wait (ms)(milliseconds to wait=u32 500) -> ()  [unwired: 1 out]
                                }
                                frame #2 {
                                n1413 = property on="Load parameters" class="Bool (strict)"("Val(Sgnl)"=TRUE ("Value (Signaling)")) -> ()  [unwired: 2 in, 2 out]
                                n1414 = case shown="True" "Green ON During Raster" {
                                frame False {
                                }
                                frame True {
                                n1415 = property on="Green Laser ON" class="Bool (strict)"("Val(Sgnl)"=TRUE ("Value (Signaling)")) -> ()  [unwired: 2 in, 2 out]
                                }
                                }
                                }
                                frame #3 {
                                n1416 = Wait (ms)(milliseconds to wait=u32 500) -> ()  [unwired: 1 out]
                                }
                                frame #4 {
                                n1417 = property on="Trap Raster Scan" class="Bool (strict)"("Val(Sgnl)"=TRUE ("Value (Signaling)")) -> ()  [unwired: 2 in, 2 out]
                                }
                                frame #5 {
                                n1418 = Wait (ms)(milliseconds to wait=u32 2000) -> ()  [unwired: 1 out]
                                }
                                frame #6 {
                                n1419 = flat-sequence {
                                tunnel: w2184 -> [w2191]
                                frame #0 {
                                n1420 = while {
                                stop <- w2187 stop-if-true
                                n1421 = local read "Raster Scanning..."() -> (w2186:bool)
                                n1422 = local read "Saving..."() -> (w2189:bool)
                                n1423 = Wait (ms)(milliseconds to wait=u32 100) -> ()  [unwired: 1 out]
                                n1424 = Not(x=w2189) -> (.not. x?=w2188:bool)
                                n1425 = Not(x=w2186) -> (.not. x?=w2185:bool)
                                n1426 = And(x=w2188, y=w2185) -> (x .and. y?=w2187:bool)
                                }
                                }
                                frame #1 {
                                n1427 = local read "Tether"() -> (w2192:bool)
                                n1428 = case shown="True" w2192 {
                                tunnel: w2191 -> [_ w2194]
                                frame False {
                                n1429 = property on="Fish for Tether" class="Bool (strict)"("Val(Sgnl)"="Fish again after \nraster break?") -> ()  [unwired: 2 in, 2 out]
                                }
                                frame True {
                                n1430 = stacked-sequence {
                                tunnel: w2194 -> [_ w2198 _ _]
                                frame #0 {
                                n1431 = property on="Trap Delta (MHz)" class="DigNum (strict)"("Val(Sgnl)"="Move to Delta 2 (MHz)") -> ()  [unwired: 2 in, 2 out]
                                n1432 = case shown="True" "Flow ON after\ntether testing?" {
                                frame False {
                                }
                                frame True {
                                n1433 = property on="Sample Channel\nFlow" class="Bool (strict)"("Val(Sgnl)"=TRUE ("Value (Signaling)")) -> ()  [unwired: 2 in, 2 out]
                                }
                                }
                                }
                                frame #1 {
                                n1434 = flat-sequence {
                                tunnel: w2198 -> [w2200]
                                frame #0 {
                                n1435 = Wait (ms)(milliseconds to wait=u32 500) -> ()  [unwired: 1 out]
                                }
                                frame #1 {
                                n1436 = case shown="\"6\"" w2200 {
                                frame Default {
                                }
                                frame "6" {
                                n1437 = property on="Green Laser ON" class="Bool (strict)"("Val(Sgnl)"=TRUE ("Green Laser ON/Interlacing")) -> ()  [unwired: 2 in, 2 out]
                                }
                                }
                                }
                                frame #2 {
                                n1438 = Wait (ms)(milliseconds to wait=u32 500) -> ()  [unwired: 1 out]
                                }
                                frame #3 {
                                n1439 = local write "Start Saving"("Save at end (5, 6)") -> ()
                                }
                                }
                                }
                                frame #2 {
                                n1440 = local read "Bead Sep. Int. Time (s)"() -> (w2206:dbl)
                                n1441 = Multiply(x=w2206, y=1000.0) -> (x*y=w2205:dbl)
                                n1442 = Wait (ms)(milliseconds to wait=w2205) -> ()  [unwired: 1 out]
                                }
                                frame #3 {
                                n1443 = property on="Remove Offset" class="Bool (strict)"("Val(Sgnl)"=TRUE ("Value (Signaling)")) -> ()  [unwired: 2 in, 2 out]
                                }
                                }
                                }
                                }
                                }
                                }
                                }
                                }
                                }
                                frame "2", Default {
                                }
                              }
                            }
                          }
                        }
                      }
                      "Tether" <- "Tether Alarm?"
                    }
                  }
                }
                frame #2 {
                  n1444 = local read "Oscillate Set 1"() -> (w2213:bool)
                  n1445 = local read "Stop All"() -> (w2211:bool)
                  n1446 = Or(x=w2213, y=w2208) -> (x .or. y?=w2210:bool)
                  n1447 = Not(x=w2210) -> (.not. x?=w2212:bool)
                  n1448 = Compound Arithmetic op=OR(w2211, w2212) -> (w2209:bool)
                }
              }
              n1449 = node-c288() -> ()  [unwired: 2 out]
            }
            n1450 = node-c288(w2043) -> ()  [unwired: 1 out]
          }
        }
      }
      event "Fl. Triggered...": Value Change {
        n1451 = event-data() -> ()  [unwired: 7 out]
        n1452 = case shown="True" "Fl. Triggered..." {
          frame False {
          }
          frame True {
            n1453 = node-c288() -> (w2224:T28)  [unwired: 4 out]
            n1454 = timed-loop {
              timing: w2224 -> [_]
              timing-out: [_] -> w2223
              tunnel: "Action" -> [w2232]
              shift-right: [w2229] -> _
              shift-left: u8 255 -> [w2231]
              shift-right: [w2226] -> _
              shift-left: 255 -> [w2228]
              stop <- w2225 stop-if-true
              # "Reset confocal spot"
              n1455 = node-c288() -> ()  [unwired: 2 out]
              n1456 = flat-sequence {
                tunnel: w2232 -> [w2252]
                tunnel: w2231 -> [w2251]
                tunnel: [w2250] -> w2230
                tunnel: w2228 -> [w2237]
                tunnel: [w2236] -> w2227
                tunnel: [w2631] -> w2225
                tunnel: w2230 -> [w2630]
                tunnel: [w2630] -> w2229
                tunnel: [w2629] -> w2226
                tunnel: w2227 -> [w2629]
                frame #0 {
                  n1457 = local read "Delta Fl. 2"() -> (w2249:dbl)
                  n1458 = local read "Delta Fl. 1"() -> (w2244:dbl)
                  n1459 = Multiply(x="Fl. Delta Thresh. (kHz)", y=1000.0) -> (x*y=w2239:dbl)
                  n1460 = Select(t=w2244, s="APD to Watch", f=w2249) -> (s? t:f=w2240:dbl)
                  n1461 = Greater?(x=w2240, y=w2239) -> (0:w2245:bool)
                  n1462 = Or(x="Force Yank", y=w2245) -> (x .or. y?=w2243:bool)
                  n1463 = And(x=w2243, y="Yank when?") -> (x .and. y?=w2241:bool)
                  n1464 = case shown="False" w2241 {
                    tunnel: w2252 -> [w2255 w2456]
                    tunnel: w2251 -> [w2257 w2452]
                    tunnel: [w2257 w2450] -> w2250
                    tunnel: w2240 -> [w2263 _]
                    tunnel: w2239 -> [w2262 _]
                    tunnel: "Force Yank" -> [w2260 _]
                    tunnel: w2237 -> [w2259 w2449]
                    tunnel: [w2258 w2449] -> w2236
                    frame False {
                      n1465 = Negate(x=w2262) -> (-x=w2254:dbl)
